vi "MT Get Axis Status.vi"(11 "AObj":u16) -> (1 "pNeg":u8, 2 "pDir":u8, 3 "pRun":u8, 4 "pZero":u8, 5 "pPos":u8, 6 "function return":i32, 7 "pMode":u8)   [LabVIEW 2014, in "MT_API.lvlib"]
doc: "MT_API INT32 __stdcall MT_Get_Axis_Status(WORD AObj,BYTE* pRun,BYTE* pDir,BYTE* pNeg,BYTE* pPos,BYTE* pZero,BYTE* pMode);"
uses:
  MT_API.lvlib
  MT_API.dll
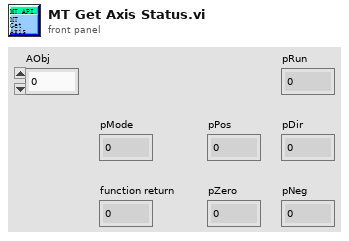
[diagram p1: front panel]
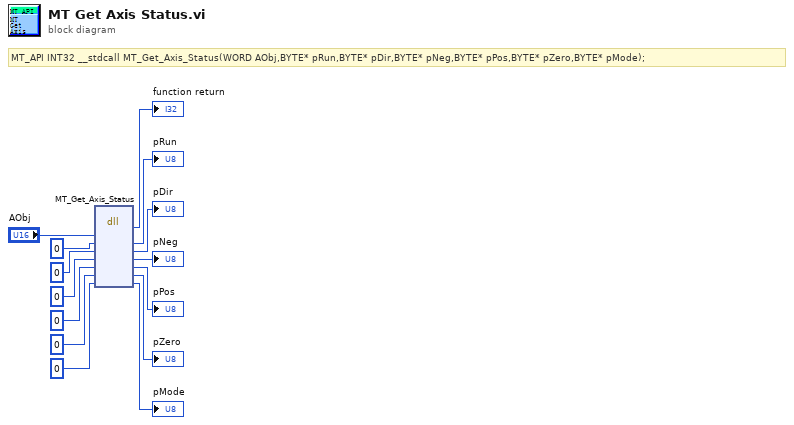
[diagram p0: block diagram]
diagram:
  # "MT_API INT32 __stdcall MT_Get_Axis_Status(WORD AObj,BYTE* pRun,BYTE* pDir,BYTE* pNeg,BYTE* pPos,BYTE* pZero,BYTE* pMode);"
  n1 = dll-call lib="E:/Projects/LabView/MT_API/MT_API.*" fn="MT_Get_Axis_Status"("AObj"="AObj", "pRun"=u8 0, "pDir"=u8 0, "pNeg"=u8 0, "pPos"=u8 0, "pZero"=u8 0, "pMode"=u8 0) -> (→"function return":i32, "pRun"=→"pRun":u8, "pDir"=→"pDir":u8, "pNeg"=→"pNeg":u8, "pPos"=→"pPos":u8, "pZero"=→"pZero":u8, "pMode"=→"pMode":u8)  [unwired: 4 in, 2 out]
